vi "BaseFolder.vi"(7 "calendarFolderTree":bool, 8 "error in (no error)":errorcluster, 9 "useUTC":bool, 10 "Timestamp":timestamp, 11 "RootFolder":path) -> (0 "error out":errorcluster, 3 "Folder":path)   [LabVIEW 2026, in "Lumberjack.lvlib"]
doc: "Pure target-folder computation. Return the folder for the current file: RootFolder, plus dated calendar subfolders when CalendarFolderTree is TRUE (SRS-LMBR-036). UseUTC selects the frame so the folder date matches the file name date. Computes the path only; folder creation happens in the sink (OpenSink). Deterministic given inputs; no I/O."
uses:
  Lumberjack.lvlib
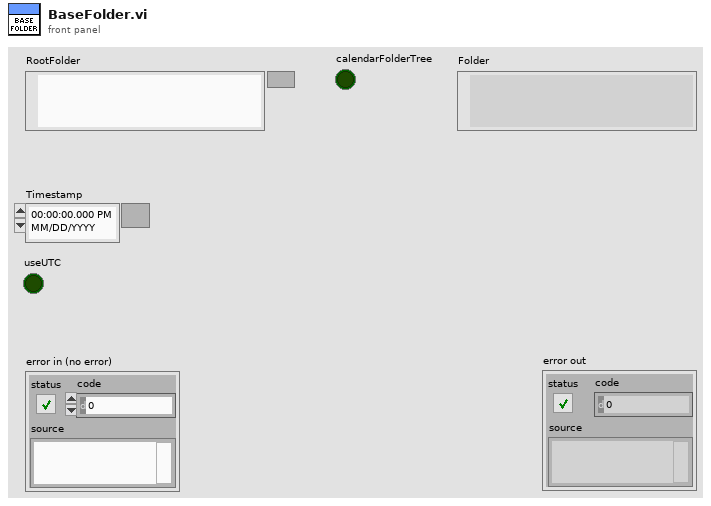
[diagram p1: front panel]
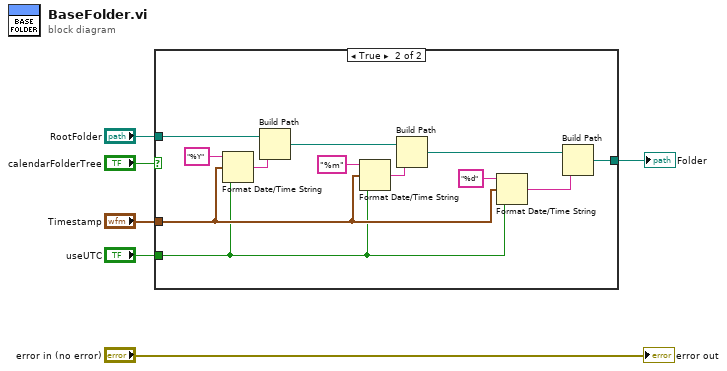
[diagram p0: block diagram]
diagram:
  n1 = case shown="True" "calendarFolderTree" {
    tunnel: "Timestamp" -> [_ w19]
    tunnel: "useUTC" -> [_ w18]
    tunnel: "RootFolder" -> [w7 w9]
    tunnel: [w7 w8] -> w1
    frame False {
    }
    frame True {
      n2 = Format Date/Time String(time format string (%c)="%Y", seconds (now)=w19, UTC format=w18) -> (date/time string=w16:string)
      n3 = Build Path(base path=w9, name or relative path=w16) -> (appended path=w11:path)
      n4 = Format Date/Time String(time format string (%c)="%m", seconds (now)=w19, UTC format=w18) -> (date/time string=w13:string)
      n5 = Build Path(base path=w11, name or relative path=w13) -> (appended path=w10:path)
      n6 = Format Date/Time String(time format string (%c)="%d", seconds (now)=w19, UTC format=w18) -> (date/time string=w12:string)
      n7 = Build Path(base path=w10, name or relative path=w12) -> (appended path=w8:path)
    }
  }
  "Folder" <- w1
  "error out" <- "error in (no error)"
